vi "Disable-Enable Button.vi"(8 "error in":errorcluster, 9 "Enabled?":bool, 10 "Refresh SRs in":refnum<vi>, 11 "Add SR in":refnum<vi>) -> (0 "error out":errorcluster, 2 "Refresh SRs out":refnum<vi>, 3 "Add SR out":refnum<vi>)   [LabVIEW 2018]
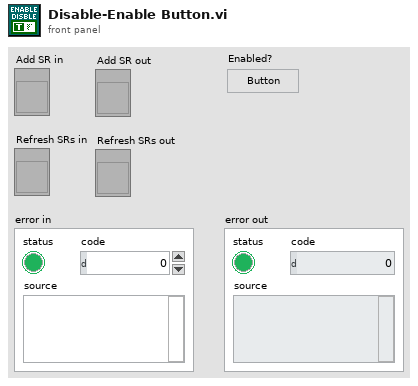
[diagram p1: front panel]
types:
  T1 = enum8{"Enabled", "Disabled", "Disabled and Grayed Out"}
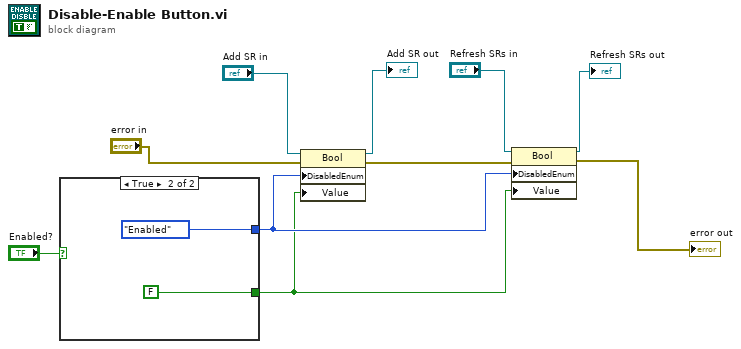
[diagram p0: block diagram]
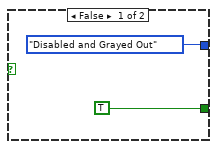
[diagram p2: hidden frame]
diagram:
  n1 = case shown="True" "Enabled?" {
    tunnel: [T1."Disabled and Grayed Out" ("Disabled") T1."Enabled" ("Disabled")] -> w2
    tunnel: [TRUE FALSE] -> w1
    frame False {
    }
    frame True {
    }
  }
  n2 = property class="Bool"(reference="Add SR in", error in="error in", "DisabledEnum"=w2, "Value"=w1) -> (reference out=→"Add SR out":refnum<vi>, error out=w5:errorcluster)
  n3 = property class="Bool"(reference="Refresh SRs in", error in=w5, "DisabledEnum"=w2, "Value"=w1) -> (reference out=→"Refresh SRs out":refnum<vi>, error out=→"error out":errorcluster)
